vi "OPC_DA_Server.vi"() -> (1 "URL":string, 2 "DA Server Running":bool, 3 "DataSocket Refnum out":refnum<k13>)   [LabVIEW 2025]
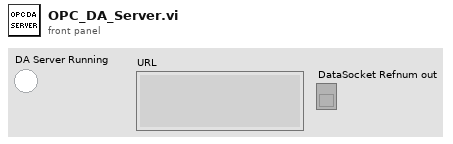
[diagram p1: front panel]
types:
  T1 = enum16{"Read", "Write", "ReadWrite", "BufferedRead", "BufferedReadWrite"}
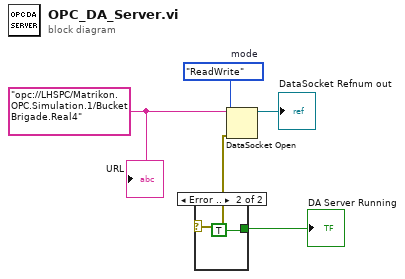
[diagram p0: block diagram]
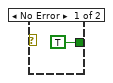
[diagram p2: hidden frame]
diagram:
  w1 = T1."ReadWrite"  # mode
  w3 = "opc://LHSPC/Matrikon.OPC.Simulation.1/Bucket Brigade.Real4"
  n1 = DataSocket Open(10:w1, 11:w3) -> (0:w4:errorcluster, 3:→"DataSocket Refnum out":refnum<k13>)  [unwired: 2 in]
  n2 = case shown="Error .." w4 {
    tunnel: [TRUE ("Server Status") TRUE ("Server Status")] -> w5
    frame No Error {
    }
    frame Error {
    }
  }
  "DA Server Running" <- w5
  "URL" <- w3
